vi "Load_from_Project.vi"(8 "error in (no error)":errorcluster, 9 "index":string, 10 "buildObject":T1, 11 "absFolder.lvclass":refnum<class "absFolder.lvclass">) -> (0 "error out":errorcluster, 1 "index out":string, 2 "buildObject out":T1, 3 "absFolder out":refnum<class "absFolder.lvclass">)   [LabVIEW 2020, in "absFolder.lvclass"]
uses:
  <vilib>/AppBuilder/IB_Classes/Destination/absFolder/absFolder.lvclass
  <vilib>/AppBuilder/IB_Classes/Destination/absFolder/absFolder.lvclass/absFolder.ctl
  <vilib>/AppBuilder/IB_Classes/Destination/IB_Destination.lvclass
  <vilib>/AppBuilder/IB_RW_Project/IB_RW_Project_PropBag_Action.ctl
  <resource>/Framework/Providers/API/ItemRef.ctl
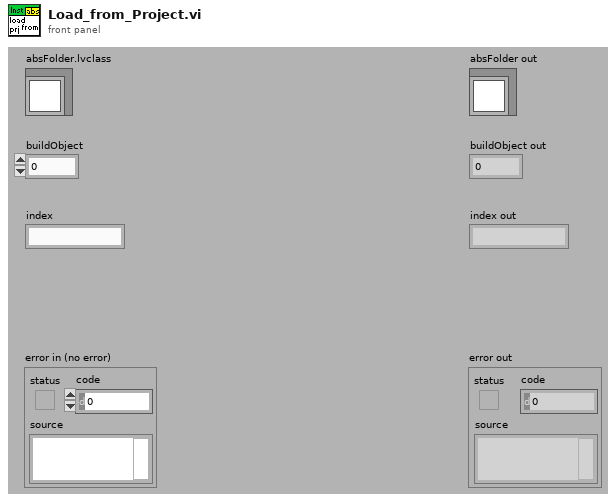
[diagram p1: front panel]
types:
  T1 = typedef "ItemRef.ctl" = u64
  T2 = typedef "IB_RW_Project_PropBag_Action.ctl" = enum16{"read", "write", "clear", "readPrevious", "writePrevious", "clearPrevious"}
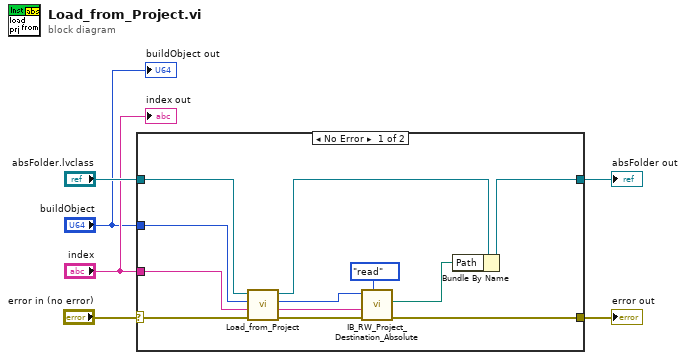
[diagram p0: block diagram]
diagram:
  n1 = case shown="No Error" "error in (no error)" {
    selector: "error in (no error)" -> [w7 w19]
    tunnel: "index" -> [w18 _]
    tunnel: "buildObject" -> [w17 _]
    tunnel: "absFolder.lvclass" -> [w16 w20]
    tunnel: [w13 w20] -> w5
    tunnel: [w10 w19] -> w4
    frame No Error {
      n2 = call-parent "Load_from_Project.vi"("error in (no error)"=w7, "index"=w18, "buildObject"=w17, "IB_Destination.lvclass"=w16) -> ("error out"=w11:errorcluster, "index out"=w8:string, "buildObject out"=w9:T1, "IB_Destination out"=w14:refnum<class "absFolder.lvclass">)  [unwired: 4 in]
      n3 = call <vilib>:"IB_RW_Project_Destination_Absolute.vi"("action"=IB_RW_Project_PropBag_Action."read", "ErrIn"=w11, "index"=w8, "buildObject"=w9) -> ("ErrOut"=w10:errorcluster, "Path"=w12:path)  [unwired: 4 in, 2 out]
      n4 = Bundle By Name(cluster=w14, "Path"=w12) -> (w13:refnum<class "absFolder.lvclass">)
    }
    frame Error {
    }
  }
  "error out" <- w4
  "absFolder out" <- w5
  "buildObject out" <- "buildObject"
  "index out" <- "index"
